vi "MainVI.vi"(8 "error in (no error)":errorcluster) -> (0 "error out":errorcluster)   [LabVIEW 2017]
uses:
  Support VIs/Globals.vi
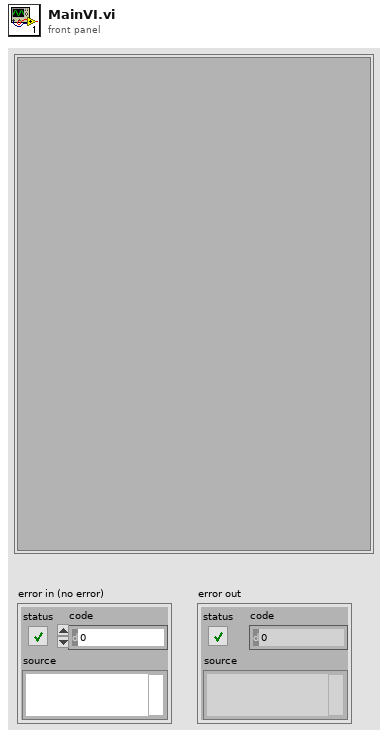
[diagram p1: front panel]
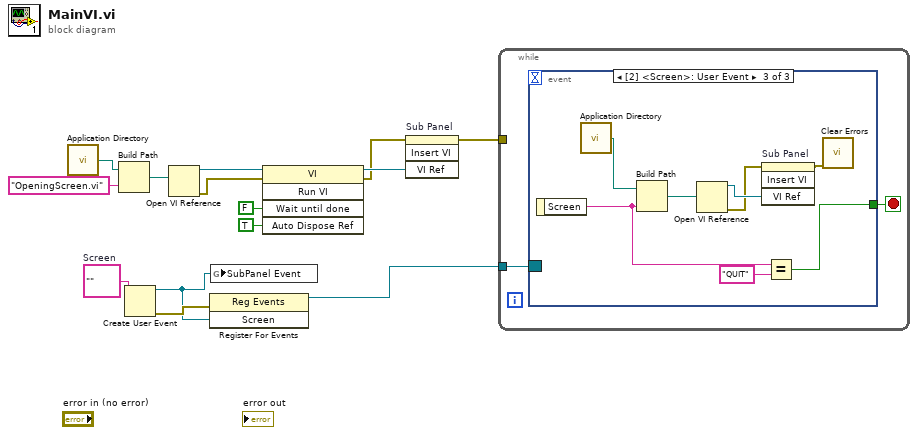
[diagram p0: block diagram]
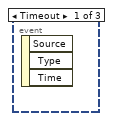
[diagram p2: hidden frame]
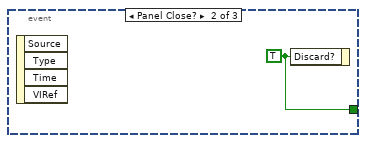
[diagram p3: hidden frame]
diagram:
  w4 = ""  # Screen
  n1 = call <vilib>:"Application Directory.vi"() -> ("Application Directory"=w14:path)
  n2 = Build Path(base path=w14, name or relative path="OpeningScreen.vi") -> (appended path=w12:path)
  n3 = Create User Event(user event datatype=w4) -> (user event=w1:refnum<user-event>, error out=w3:errorcluster)  [unwired: 1 in]
  n4 = Open VI Reference(vi path=w12) -> (vi reference=w11:refnum<vi>, error out=w7:errorcluster)  [unwired: 5 in]
  n5 = register-events(error in=w3, w1) -> (reference out=w2:refnum<event-registration>)  [unwired: 1 in, 1 out]
  n6 = global write "Globals.vi" "SubPanel Event"(w1) -> ()
  n7 = invoke class="VI" method="Run VI"(reference=w11, error in=w7, "Wait until done"=FALSE ("Wait Until Done"), "Auto Dispose Ref"=TRUE ("Auto Dispose Reference")) -> (reference out=w10:refnum<vi>, error out=w6:errorcluster)  [unwired: 1 in, 3 out]
  n8 = invoke on="Sub Panel" class="SubPnl" method="Insert VI"(error in=w6, "VI Ref"=w10) -> (error out=w5:errorcluster)  [unwired: 2 in, 3 out]
  n9 = while {
    tunnel: w5 -> [_]
    tunnel: w2 -> [w15]
    stop <- w16 stop-if-true
    n10 = event shown="[2] <Screen>: User Event" {
      selector: w15 -> [_ _ _]
      dyn-events: _ -> [_ _ _]
      timeout: _ -> [_ _ _]
      tunnel: [_ w17 w20] -> w16
      event Timeout {
        n11 = event-data() -> ()  [unwired: 1 in, 3 out]
      }
      event Panel Close? {
        w17 = TRUE ("Discard?")
        n12 = event-data() -> ()  [unwired: 1 in, 4 out]
        n13 = event-data("Discard?"=w17) -> ()  [unwired: 1 in, 1 out]
      }
      event User Event {
        n14 = event-data() -> ("Screen"=w22:string)  [unwired: 1 in]
        n15 = call <vilib>:"Application Directory.vi"() -> ("Application Directory"=w25:path)
        n16 = Build Path(base path=w25, name or relative path=w22) -> (appended path=w24:path)
        n17 = Open VI Reference(vi path=w24) -> (vi reference=w23:refnum<vi>, error out=w18:errorcluster)  [unwired: 5 in]
        n18 = invoke on="Sub Panel" class="SubPnl" method="Insert VI"(error in=w18, "VI Ref"=w23) -> (error out=w19:errorcluster)  [unwired: 2 in, 3 out]
        n19 = Equal?(x=w22, y="QUIT") -> (x = y?=w20:bool)
        n20 = call <vilib>:"Clear Errors.vi"("error in (no error)"=w19) -> ()  [unwired: 5 in, 2 out]
      }
    }
  }
